vi "y1y2 (子VI).vi"(5 "二值化输入":u8[][](array[numeric]), 7 "Image Pixels (U8)输入":u8[][](array[numeric])) -> (0 "添加的数组":cluster{i32, i32}[](array[cluster]), 2 "四个角点":i32[][](array[numeric]))   [LabVIEW 2014]
panel:
  # "x"
  # "1"
  # "2"
  # "y"
  # "x"
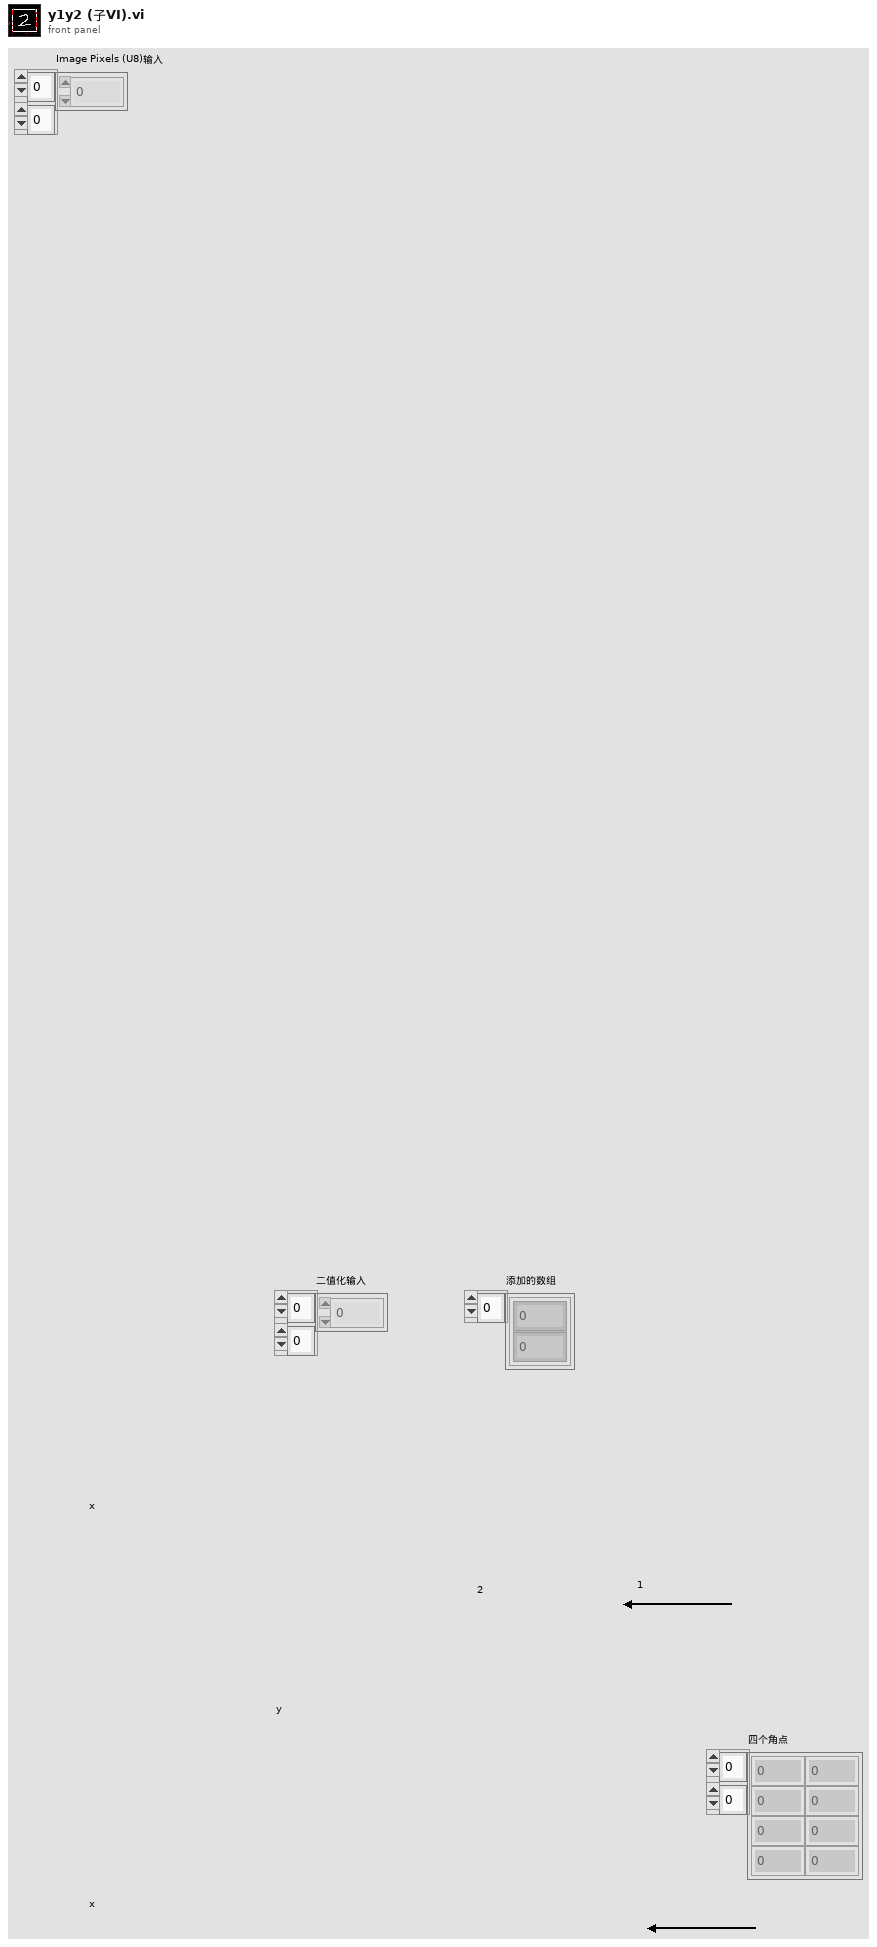
[diagram p1: front panel]
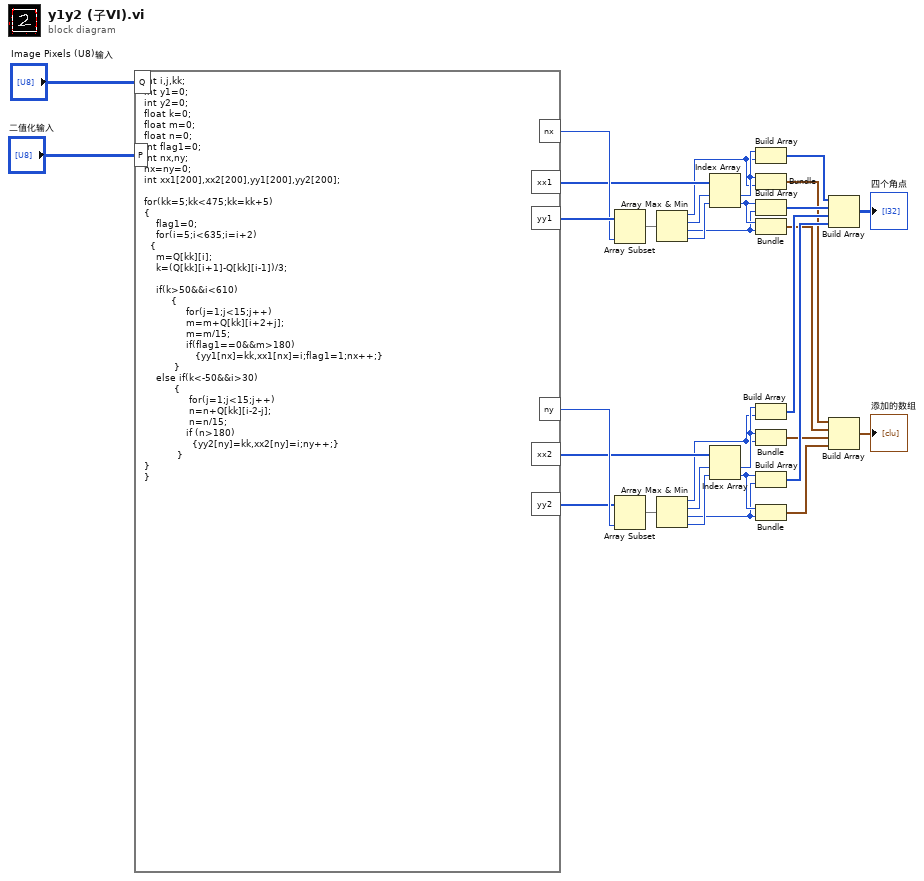
[diagram p0: block diagram]
diagram:
  n1 = formula code="int i,j,kk;\nint y1=0;\nint y2=0;\nfloat k=0;\nfloat m=0;\nfloat n=0;\nint flag1=0;\nint nx,ny;\nnx=ny=0;\nint xx1[200],xx2[200],yy1[200],yy2[200];\n\nfor(kk=5;kk<475;kk=kk+5)\n{\n    flag1=0;\n    for(i=5;i<635;i=i+2)\n  {\n    m=Q[kk][i];\n    k=(Q[kk][i+1]-Q[kk][i-1])/3;\n\n    if(k>50&&i<610)\n         {   \n              for(j=1;j<15;j++)\n              m=m+Q[kk][i+2+j];\n              m=m/15;\n              if(flag1==0&&m>180)\n                 {yy1[nx]=kk,xx1[nx]=i;flag1=1;nx++;}\n          }\n    else if(k<-50&&i>30)\n          {                   \n               for(j=1;j<15;j++)\n               n=n+Q[kk][i-2-j];\n               n=n/15;\n              if (n>180)\n                {yy2[ny]=kk,xx2[ny]=i;ny++;}\n           }\n}\n}"("Q"="Image Pixels (U8)输入", "P"="二值化输入") -> ("xx1"=w25:i32[], "yy1"=w32:i32[], "nx"=w31:i32, "xx2"=w19:i32[], "yy2"=w29:i32[], "ny"=w30:i32)
  n2 = Array Subset(array=w32, length=w31) -> (w27:i32[])  [unwired: 1 in]
  n3 = Array Subset(array=w29, length=w30) -> (w26:i32[])  [unwired: 1 in]
  n4 = Array Max & Min(array=w27) -> (max value=w12:i32, max index (indices)=w24:i32, min value=w10:i32, min index (indices)=w23:i32)
  n5 = Array Max & Min(array=w26) -> (max value=w8:i32, max index (indices)=w18:i32, min value=w6:i32, min index (indices)=w17:i32)
  n6 = Index Array(array=w25, index #1=w24, index #2=w23) -> (element #1=w13:i32, element #2=w11:i32)
  n7 = Index Array(array=w19, index #1=w18, index #2=w17) -> (element #1=w9:i32, element #2=w7:i32)
  n8 = Build Array(w13, w12) -> (w22:i32[])
  n9 = Bundle(w13, w12) -> (w5:cluster{i32, i32})  [unwired: 1 in]
  n10 = Build Array(w11, w10) -> (w21:i32[])
  n11 = Bundle(w11, w10) -> (w4:cluster{i32, i32})  [unwired: 1 in]
  n12 = Build Array(w9, w8) -> (w16:i32[])
  n13 = Bundle(w9, w8) -> (w3:cluster{i32, i32})  [unwired: 1 in]
  n14 = Build Array(w7, w6) -> (w15:i32[])
  n15 = Bundle(w7, w6) -> (w2:cluster{i32, i32})  [unwired: 1 in]
  n16 = Build Array(w22, w21, w16, w15) -> (→"四个角点":i32[][])
  n17 = Build Array(w5, w4, w3, w2) -> (→"添加的数组":cluster{i32, i32}[])
